vi "ADIS16448-Teensy Example.vi"() -> ()   [LabVIEW 2016]
uses:
  ADIS16448-Teensy/ADIS16448-Teensy.lvlib
panel:
  in  "Z Orientation":enum16{"Z Up", "Z Down"}(ring)=enum."Z Down"
  out "IMU AHRS Out":cluster{"Pitch":dbl, "Roll":dbl, "Yaw":dbl} {"Roll" scale=-180.0..180.0; "Pitch" scale=-90.0..90.0}
  out "IMU Angles Out":cluster{"X":dbl, "Y":dbl, "Z":dbl} {"X" scale=-180.0..180.0; "Y" scale=-180.0..180.0; "Z" scale=-180.0..180.0}
  in  "Reset":bool
  out "IMU AHRS Out":cluster{"Pitch":dbl, "Roll":dbl, "Yaw":dbl}
  out "IMU Angles Out":T1
  in  "stop":bool
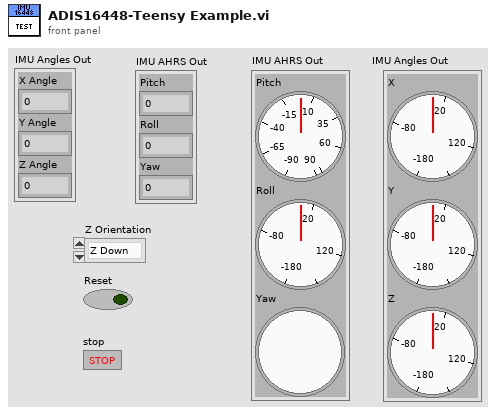
[diagram p1: front panel]
types:
  T1 = cluster{"X Angle":dbl, "Y Angle":dbl, "Z Angle":dbl}
  T2 = typedef "WPI_SerialPortRef.ctl" = cluster{"DevStatus":errorcluster, "Serial Port Name":refnum<visa-resource-name>}
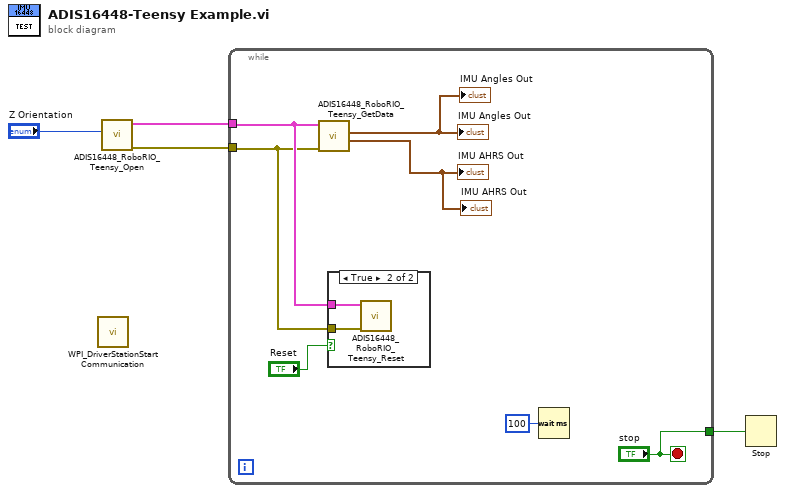
[diagram p0: block diagram]
diagram:
  n1 = call <vilib>:"WPI_DriverStationStart Communication.vi"() -> ()  [unwired: 12 in]
  n2 = call "ADIS16448_RoboRIO_Teensy_Open.vi"("Z Orientation"="Z Orientation") -> ("error out"=w3:errorcluster, "SerialPortRef"=w4:T2)  [unwired: 8 in]
  n3 = while {
    tunnel: w4 -> [w9]
    tunnel: w3 -> [w8]
    tunnel: ["stop"] -> w2
    stop <- "stop" stop-if-true
    n4 = call "ADIS16448_RoboRIO_Teensy_GetData.vi"("error in"=w8, "SerialPortRefIn"=w9) -> ("IMU AHRS Out"=→"IMU AHRS Out" →"IMU AHRS Out":cluster{"Pitch":dbl, "Roll":dbl, "Yaw":dbl}, "IMU Angles Out"=→"IMU Angles Out" →"IMU Angles Out":T1)  [unwired: 6 in, 2 out]
    n5 = case shown="True" "Reset" {
      tunnel: w9 -> [_ w13]
      tunnel: w8 -> [_ w12]
      frame False {
      }
      frame True {
        n6 = call "ADIS16448_RoboRIO_Teensy_Reset.vi"("error in"=w12, "SerialPortRef"=w13) -> ()  [unwired: 8 in, 2 out]
      }
    }
    n7 = Wait (ms)(milliseconds to wait=u32 100) -> ()  [unwired: 1 out]
  }
  n8 = Stop(stop? (T)=w2) -> ()
